vi "Load Modules.vi"(8 "error in (no error)":errorcluster, 11 "Application Controller in":refnum<class "Application Controller.lvclass">) -> (0 "error out":errorcluster, 3 "Application Controller out":refnum<class "Application Controller.lvclass">)   [LabVIEW 2020, in "Application Controller.lvclass"]
uses:
  Application Controller.lvclass
  opt/github/LabActor/Template Module/Template Module.lvclass
  Menu Control.ctl
  Monitor Controller/Monitor Controller.lvclass
  Recorders/PID Controller/PID Controller.lvclass
  Recorders/VI Server/VI Server Recorder.lvclass
  Post-Processors/Lockin Processor/Lockin Processor.lvclass
  Comms/TCP Communications/TCP Communications.lvclass
  Template Module/Template Module.lvclass/Template Module.ctl
  Application Controller.lvclass/Application Controller.ctl
  Template Module/Read Name.vi
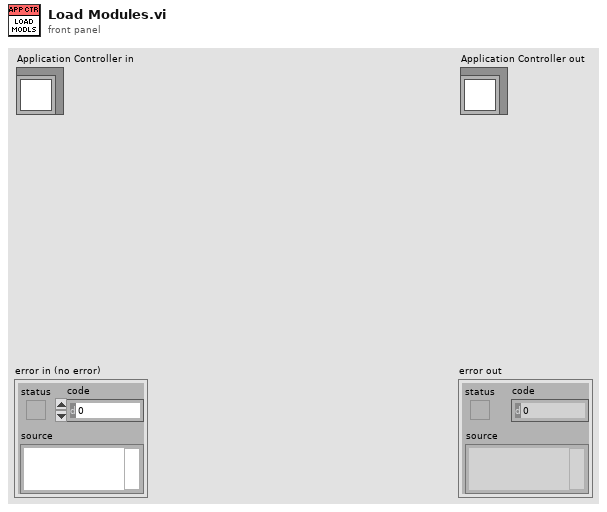
[diagram p1: front panel]
types:
  T1 = typedef "Menu Control.ctl" = enum16{"NONE", "Monitor", "Post-process", "Pulse"}
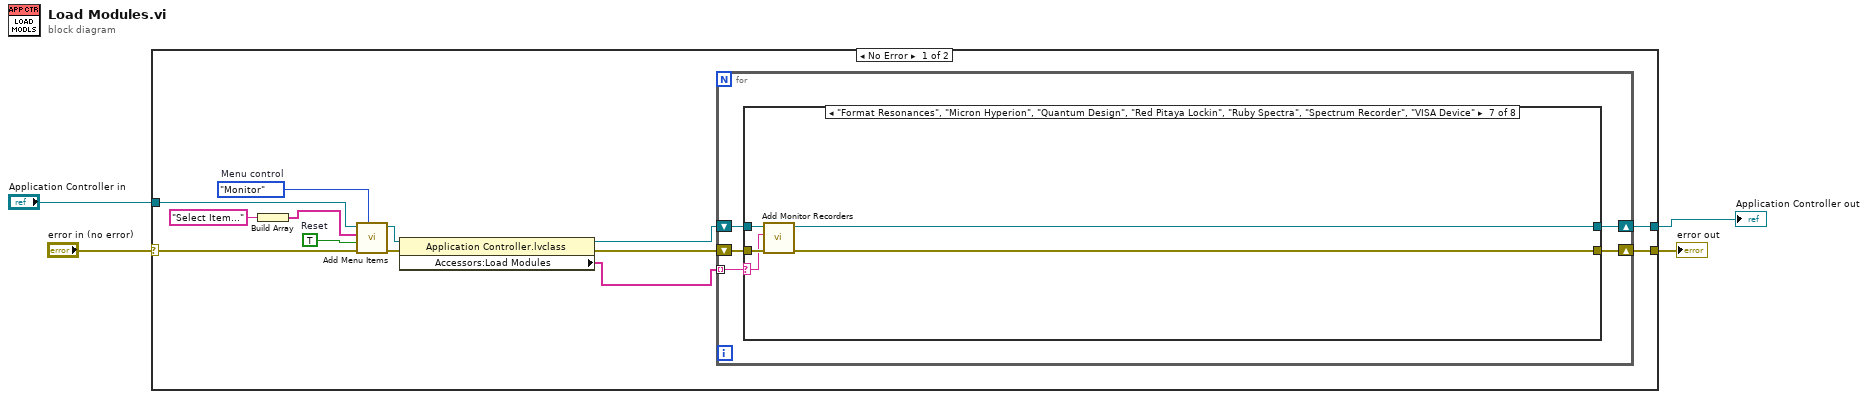
[diagram p0: block diagram]
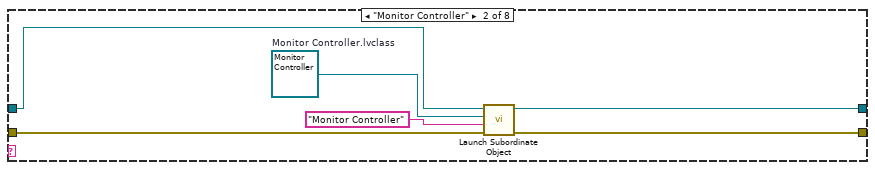
[diagram p3: hidden frame]
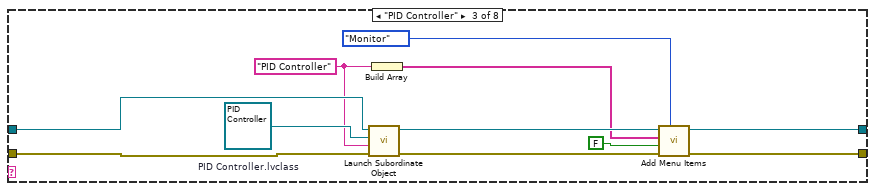
[diagram p4: hidden frame]
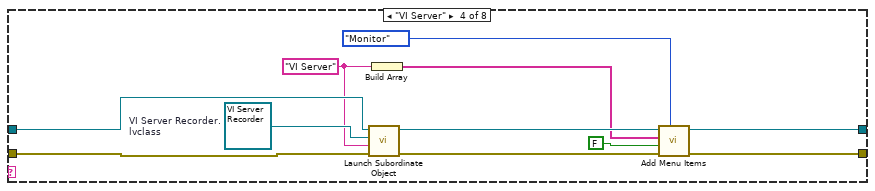
[diagram p5: hidden frame]
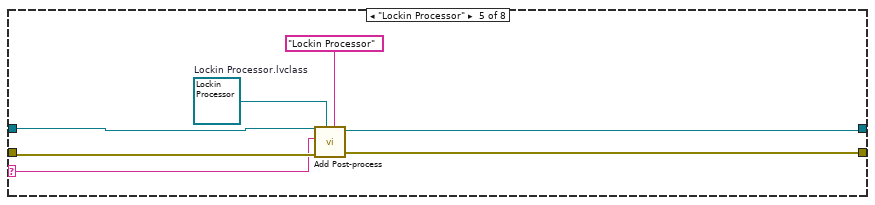
[diagram p6: hidden frame]
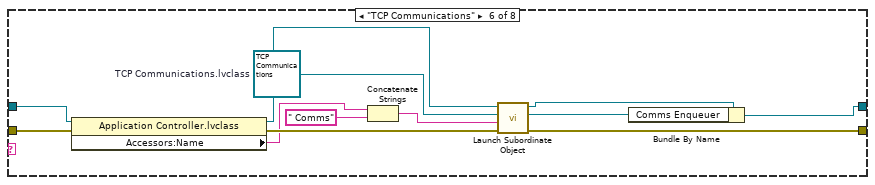
[diagram p7: hidden frame]
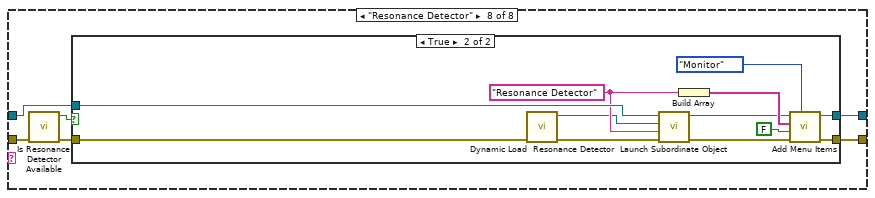
[diagram p8: hidden frame]
diagram:
  n1 = case shown="No Error" "error in (no error)" {
    selector: "error in (no error)" -> [w9 w98]
    tunnel: [w14 w98] -> w3
    tunnel: [w15 w97] -> w1
    tunnel: "Application Controller in" -> [w6 w97]
    frame No Error {
      w8 = Menu_Control."Monitor"  # Menu control
      w12 = TRUE  # Reset
      n2 = Build Array("Select Item..." ("element")) -> (w13:string[])
      n3 = call-dynamic "Add Menu Items.vi"("Menu control"=w8, "error in (no error)"=w9, "Reset"=w12, "Item Names"=w13, "Application Controller in"=w6) -> ("error out"=w10:errorcluster, "Application Controller out"=w7:refnum<class "Application Controller.lvclass">)  [unwired: 5 in]
      n4 = property class="Application Controller.lvclass"(reference=w7, error in=w10) -> (reference out=w17:refnum<class "Application Controller.lvclass">, error out=w16:errorcluster, "Accessors:Load Modules"=w5:string[])
      n5 = for {
        tunnel: w5 -> [w22] mode=indexing
        shift-right: [w20] -> w14
        shift-left: w16 -> [w21]
        shift-right: [w19] -> w15
        shift-left: w17 -> [w18]
        n6 = case shown="\"Format Resonances\", \"Micron Hyperion\", \"Quantum Design\", \"Red Pitaya Lockin\", \"Ruby Spectra\", \"Spectrum Recorder\", \"VISA Device\"" w22 {
          selector: w22 -> [_ _ _ _ w53 _ w72 _]
          tunnel: w21 -> [w23 w28 w40 w51 w54 w70 w76 w78]
          tunnel: [w23 w27 w34 w45 w55 w69 w75 w81] -> w20
          tunnel: w18 -> [w24 w30 w41 w52 w57 w66 w74 w82]
          tunnel: [w24 w29 w35 w46 w56 w61 w73 w80] -> w19
          frame "NONE", Default {
          }
          frame "Monitor Controller" {
            w26 = refnum<class "Monitor Controller.lvclass"> refnum  # Monitor Controller.lvclass
            n7 = call-dynamic "Launch Subordinate Object.vi"("error in (no error)"=w28, "Name"="Monitor Controller", "Subordinate Object"=w26, "Application Controller in"=w30) -> ("error out"=w27:errorcluster, "Application Controller out"=w29:refnum<class "Application Controller.lvclass">)  [unwired: 5 in, 1 out]
          }
          frame "PID Controller" {
            w32 = "PID Controller" ("Name")
            w39 = refnum<class "PID Controller.lvclass"> refnum  # PID Controller.lvclass
            n8 = call-dynamic "Launch Subordinate Object.vi"("error in (no error)"=w40, "Name"=w32, "Subordinate Object"=w39, "Application Controller in"=w41) -> ("error out"=w33:errorcluster, "Application Controller out"=w36:refnum<class "Application Controller.lvclass">)  [unwired: 5 in, 1 out]
            n9 = Build Array(w32) -> (w31:string[])
            n10 = call-dynamic "Add Menu Items.vi"("Menu control"=Menu_Control."Monitor", "error in (no error)"=w33, "Reset"=FALSE, "Item Names"=w31, "Application Controller in"=w36) -> ("error out"=w34:errorcluster, "Application Controller out"=w35:refnum<class "Application Controller.lvclass">)  [unwired: 5 in]
          }
          frame "VI Server" {
            w43 = "VI Server" ("Name")
            w50 = refnum<class "VI Server Recorder.lvclass"> refnum  # VI Server Recorder.lvclass
            n11 = call-dynamic "Launch Subordinate Object.vi"("error in (no error)"=w51, "Name"=w43, "Subordinate Object"=w50, "Application Controller in"=w52) -> ("error out"=w44:errorcluster, "Application Controller out"=w47:refnum<class "Application Controller.lvclass">)  [unwired: 5 in, 1 out]
            n12 = Build Array(w43) -> (w42:string[])
            n13 = call-dynamic "Add Menu Items.vi"("Menu control"=Menu_Control."Monitor", "error in (no error)"=w44, "Reset"=FALSE, "Item Names"=w42, "Application Controller in"=w47) -> ("error out"=w45:errorcluster, "Application Controller out"=w46:refnum<class "Application Controller.lvclass">)  [unwired: 5 in]
          }
          frame "Lockin Processor" {
            w58 = refnum<class "Lockin Processor.lvclass"> refnum  # Lockin Processor.lvclass
            n14 = call-dynamic "Add Post-process.vi"("Name"="Lockin Processor", "Subordinate Object"=w58, "error in (no error)"=w54, "String"=w53, "Application Controller in"=w57) -> ("error out"=w55:errorcluster, "Application Controller out"=w56:refnum<class "Application Controller.lvclass">)  [unwired: 5 in]
          }
          frame "TCP Communications" {
            w68 = refnum<class "TCP Communications.lvclass"> refnum  # TCP Communications.lvclass
            n15 = property class="Application Controller.lvclass"(reference=w66, error in=w70) -> (reference out=w65:refnum<class "Application Controller.lvclass">, error out=w67:errorcluster, "Accessors:Name"=w64:string)
            n16 = Concatenate Strings(w64, " Comms" ("Name")) -> (w62:string)
            n17 = call-dynamic "Launch Subordinate Object.vi"("error in (no error)"=w67, "Name"=w62, "Subordinate Object"=w68, "Application Controller in"=w65) -> ("error out"=w69:errorcluster, "Nested Actor's Enqueuer"=w60:refnum<class "Message Enqueuer.lvclass">, "Application Controller out"=w71:refnum<class "Application Controller.lvclass">)  [unwired: 5 in]
            n18 = Bundle By Name(cluster=w71, "Comms Enqueuer"=w60) -> (w61:refnum<class "Application Controller.lvclass">)
          }
          frame "Format Resonances", "Micron Hyperion", "Quantum Design", "Red Pitaya Lockin", "Ruby Spectra", "Spectrum Recorder", "VISA Device" {
            n19 = call-dynamic "Add Monitor Recorders.vi"("error in (no error)"=w76, "String"=w72, "Application Controller in"=w74) -> ("error out"=w75:errorcluster, "Application Controller out"=w73:refnum<class "Application Controller.lvclass">)  [unwired: 6 in, 1 out]
          }
          frame "Resonance Detector" {
            n20 = call "Is Resonance Detector Available.vi"("Error In"=w78) -> ("Error Out"=w77:errorcluster, "Good"=w79:bool)  [unwired: 8 in, 1 out]
            n21 = case shown="True" w79 {
              tunnel: w77 -> [w83 w87]
              tunnel: w82 -> [w84 w96]
              tunnel: [w83 w92] -> w81
              tunnel: [w84 w89] -> w80
              frame False {
              }
              frame True {
                w95 = "Resonance Detector" ("Name")
                n22 = call "Dynamic Load  Resonance Detector.vi"("Error In"=w87) -> ("Error Out"=w86:errorcluster, "Module"=w85:refnum<class "Template Module.lvclass">)  [unwired: 9 in]
                n23 = call-dynamic "Launch Subordinate Object.vi"("error in (no error)"=w86, "Name"=w95, "Subordinate Object"=w85, "Application Controller in"=w96) -> ("error out"=w93:errorcluster, "Application Controller out"=w90:refnum<class "Application Controller.lvclass">)  [unwired: 5 in, 1 out]
                n24 = Build Array(w95) -> (w94:string[])
                n25 = call-dynamic "Add Menu Items.vi"("Menu control"=Menu_Control."Monitor", "error in (no error)"=w93, "Reset"=FALSE, "Item Names"=w94, "Application Controller in"=w90) -> ("error out"=w92:errorcluster, "Application Controller out"=w89:refnum<class "Application Controller.lvclass">)  [unwired: 5 in]
              }
            }
          }
        }
      }
    }
    frame Error {
    }
  }
  "error out" <- w3
  "Application Controller out" <- w1
